vi "sutter driver.vi"(5 "Motor":i32, 6 "error in":errorcluster, 7 "Motor Poisition":cluster{"Go Home":bool, "Position":dbl[]}, 8 "Data Change":bool, 9 "VISA resource In":refnum<visa-resource-name>) -> (0 "error out":errorcluster, 2 "VISA resource name out":refnum<visa-resource-name>)   [LabVIEW 2016]
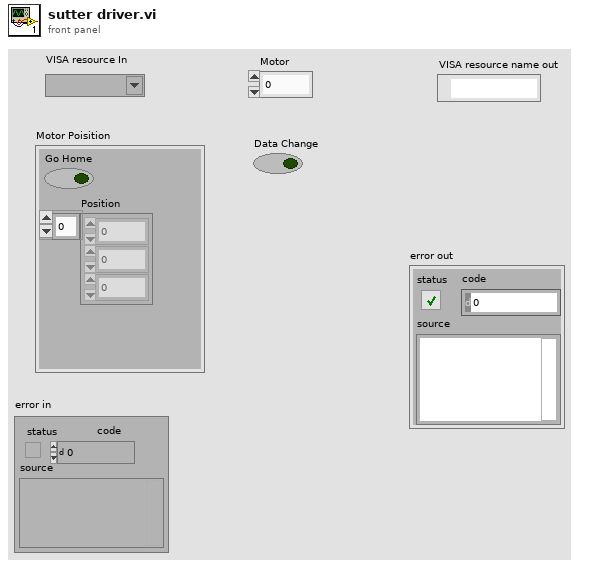
[diagram p1: front panel]
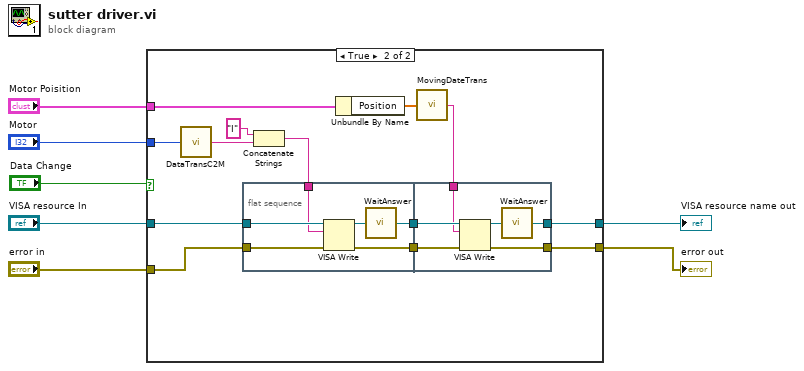
[diagram p0: block diagram]
diagram:
  n1 = case shown="True" "Data Change" {
    tunnel: [w9 w20] -> w7
    tunnel: [w8 w19] -> w6
    tunnel: "VISA resource In" -> [w9 w18]
    tunnel: "error in" -> [w8 w17]
    tunnel: "Motor" -> [_ w16]
    tunnel: "Motor Poisition" -> [_ w10]
    frame False {
    }
    frame True {
      n2 = call "DataTransC2M.vi"("input"=w16) -> ("output"=w13:string)
      n3 = flat-sequence {
        tunnel: w18 -> [w25]
        tunnel: w17 -> [w28]
        tunnel: [w27] -> w22
        tunnel: [w26] -> w21
        tunnel: w12 -> [w23]
        tunnel: w22 -> [w33]
        tunnel: w21 -> [w32]
        tunnel: [w31] -> w20
        tunnel: [w30] -> w19
        tunnel: w11 -> [w29]
        frame #0 {
          n4 = VISA Write(VISA resource name=w25, write buffer=w23, error in (no error)=w28) -> (VISA resource name out=w24:refnum<visa-resource-name>, error out=w26:errorcluster)  [unwired: 1 out]
          n5 = call "WaitAnswer.vi"("VISA resource name in"=w24) -> ("VISA resource name out"=w27:refnum<visa-resource-name>)
        }
        frame #1 {
          n6 = VISA Write(VISA resource name=w33, write buffer=w29, error in (no error)=w32) -> (VISA resource name out=w34:refnum<visa-resource-name>, error out=w30:errorcluster)  [unwired: 1 out]
          n7 = call "WaitAnswer.vi"("VISA resource name in"=w34) -> ("VISA resource name out"=w31:refnum<visa-resource-name>)
        }
      }
      n8 = Concatenate Strings("I" ("string"), w13) -> (w12:string)
      n9 = Unbundle By Name(w10) -> ("Position"=w15:dbl[])
      n10 = call "MovingDateTrans.vi"("INPUT"=w15) -> ("MOVEING COMMAND"=w11:string)  [unwired: 2 in]
    }
  }
  "error out" <- w6
  "VISA resource name out" <- w7
